vi "rearrange_controls.vi"(8 "error in":errorcluster, 10 "Ctrl Sequences":string[](array[string]), 11 "vi reference in":refnum<vi>) -> (0 "error out":errorcluster, 3 "vi reference out":refnum<vi>)   [LabVIEW 2018]
uses:
  Common/VI Scripting/VI/Front Panel/Front Panel.lvlib
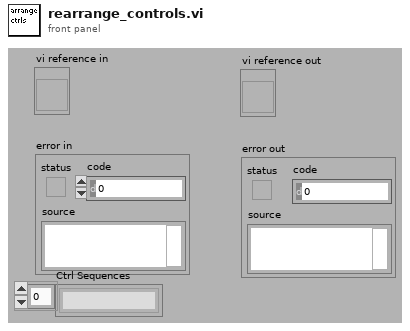
[diagram p1: front panel]
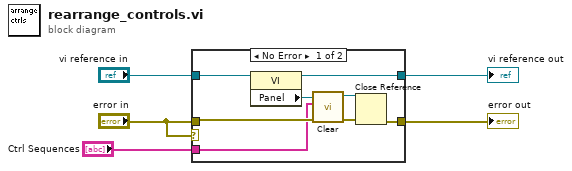
[diagram p0: block diagram]
diagram:
  n1 = case shown="No Error" "error in" {
    tunnel: [w13 w15] -> w5
    tunnel: "vi reference in" -> [w12 w14]
    tunnel: "error in" -> [w7 w15]
    tunnel: [w11 w14] -> w3
    tunnel: "Ctrl Sequences" -> [w6 _]
    frame No Error {
      n2 = property class="VI"(reference=w12) -> (reference out=w11:refnum<vi>, "Panel"=w9:refnum<vi>)  [unwired: 1 in, 1 out]
      n3 = call "Clear.vi"("error in (no error)"=w7, "Ctrl Sequences"=w6, "front panel"=w9) -> ("error out"=w10:errorcluster, "front panel out"=w8:refnum<vi>)  [unwired: 7 out]
      n4 = Close Reference(reference=w8, error in (no error)=w10) -> (error out=w13:errorcluster)
    }
    frame Error {
    }
  }
  "error out" <- w5
  "vi reference out" <- w3
